vi "H5Dopen.vi"(6 "error in (no error)":errorcluster, 7 "dapl_id":T1, 8 "name":string, 9 "HDF5 Ref":T1) -> (0 "error out":errorcluster, 2 "HDF5 Dataset Ref":T1, 3 "HDF5 Ref out":T1)   [LabVIEW 2017]
doc: "Opens an existing dataset."
uses:
  <vilib>/UPVI/lvhdf5/library.llb/HDF5 Ref.ctl
  <vilib>/UPVI/lvhdf5/hdf5.dll
panel:
  # "LVHDF5 Toolkit\nCopyright (c) 2005-2013 by Jason D. Sommerville\nCopyright (c) 2014 by UPVI, LLC.\n\nThis use and distribution of this file is governed by the terms found in \nLICENSE.txt distributed with this toolkit and installed at\n <user.lib>\\_lvhdf5\\LICENSE.txt"
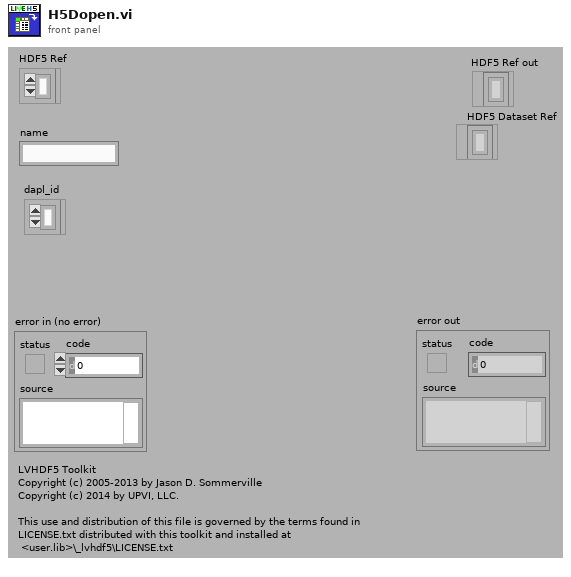
[diagram p1: front panel]
types:
  T1 = typedef "HDF5 Ref.ctl" = refnum<k1>
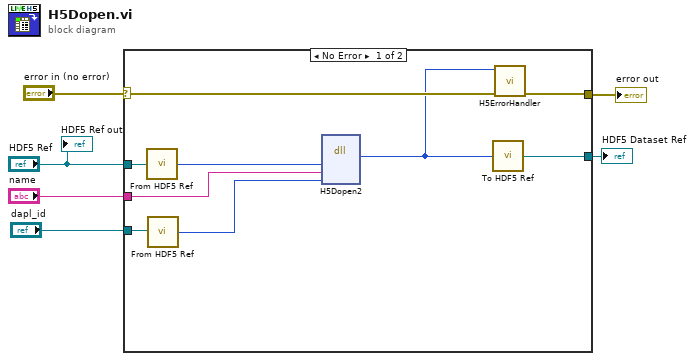
[diagram p0: block diagram]
diagram:
  n1 = case shown="No Error" "error in (no error)" {
    selector: "error in (no error)" -> [w15 w16]
    tunnel: [w14 w16] -> w5
    tunnel: "HDF5 Ref" -> [w13 _]
    tunnel: "name" -> [w11 _]
    tunnel: [w9 _] -> w2
    tunnel: "dapl_id" -> [w8 _]
    frame No Error {
      n2 = call <vilib>:"From HDF5 Ref.vi"("HDF5 Ref"=w13) -> ("I32"=w12:i32)
      n3 = call <vilib>:"From HDF5 Ref.vi"("HDF5 Ref"=w8) -> ("I32"=w7:i32)
      n4 = dll-call lib="C:/Program Files/National Instruments/LabVIEW 2017/vi.lib/UPVI/lvhdf5/hdf5.dll" fn="H5Dopen2" label="H5Dopen"("loc_id"=w12, "name"=w11, "dapl_id"=w7) -> ("return type"=w10:i32)  [unwired: 6 in, 2 out]
      n5 = call <vilib>:"To HDF5 Ref.vi"("I32"=w10) -> ("HDF5 Ref"=w9:T1)
      n6 = call <vilib>:"H5ErrorHandler.vi"("error in (no error)"=w15, "herr_t"=w10) -> ("error out"=w14:errorcluster)  [unwired: 3 in, 4 out]
    }
    frame Error {
    }
  }
  "error out" <- w5
  "HDF5 Dataset Ref" <- w2
  "HDF5 Ref out" <- "HDF5 Ref"
